vi "AutoDraw_Picture.vi"(7 "color(black)":u32(colorbox) caption="颜色（黑色）", 9 "Data Array for Picture":dbl[][](array[numeric]), 11 "Init Picture":picture) -> (2 "Anto Drawer":picture)   [LabVIEW 2014]
doc: "画平面图"
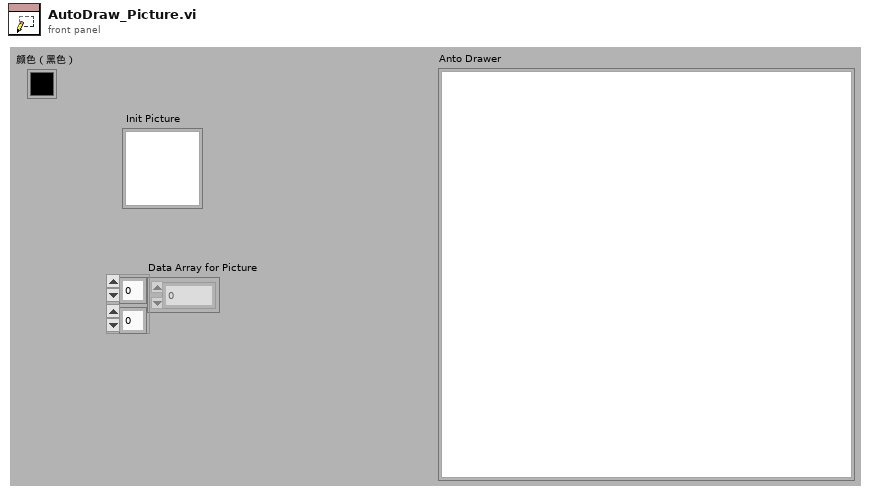
[diagram p1: front panel]
types:
  T1 = cluster{"Width":u16, "Style":enum32{"Solid", "Dash", "Dot", "DashDot", "DashDotDot"}}
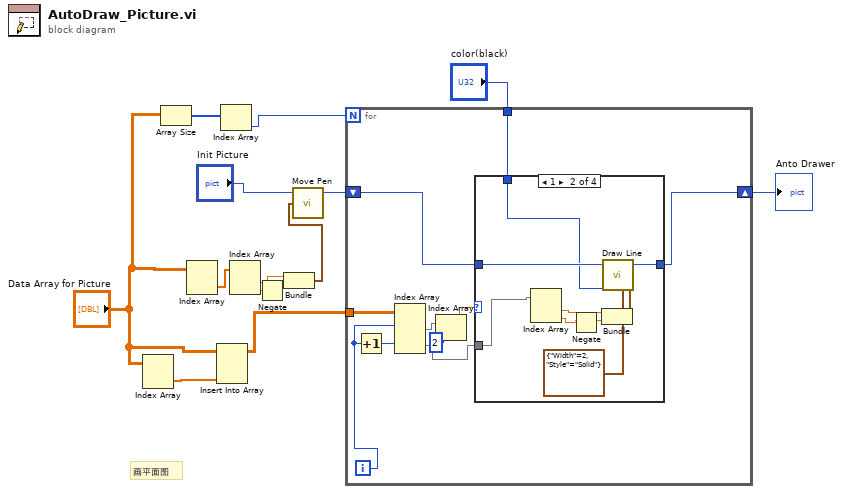
[diagram p0: block diagram]
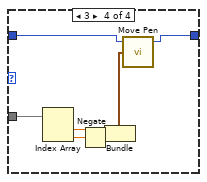
[diagram p4: hidden frame]
diagram:
  # "画平面图"
  n1 = Index Array(array="Data Array for Picture") -> (element=w7:dbl[])  [unwired: 2 in]
  n2 = Array Size(array="Data Array for Picture") -> (size(s)=w5:i32[])
  n3 = Index Array(array="Data Array for Picture") -> (element=w12:dbl[])  [unwired: 2 in]
  n4 = Insert Into Array(array="Data Array for Picture", new element=w7) -> (w6:dbl[][])  [unwired: 2 in]
  n5 = Index Array(array=w5) -> (element=w3:i32)  [unwired: 1 in]
  n6 = Index Array(array=w12) -> (element #1=w13:dbl, element #2=w14:dbl)  [unwired: 2 in]
  n7 = Negate(x=w14) -> (-x=w1:dbl)
  n8 = Bundle("x"=w13, w1) -> (w10:cluster{"x":dbl, dbl})  [unwired: 1 in]
  n9 = call <vilib>:"Move Pen.vi"("new position"=w10, "picture"="Init Picture") -> ("new picture"=w9:picture)  [unwired: 3 in]
  n10 = for {
    N: w3 -> [_]
    tunnel: w6 -> [w24]
    shift-right: [w16] -> w8
    shift-left: w9 -> [w20]
    tunnel: "color(black)" -> [w15]
    i -> [w18]
    n11 = Increment(x=w18) -> (x+1=w19:i32)
    n12 = Index Array(array=w24, index (row) #1=w18, index (row) #2=w19) -> (element #1=w21:dbl[], element #2=w17:dbl[])  [unwired: 2 in]
    n13 = Index Array(array=w21, index=2 ("索引")) -> (element=w22:dbl)
    n14 = case shown="1" w22 {
      tunnel: w20 -> [w25 w31 w35 w38]
      tunnel: [w25 w30 w35 w37] -> w16
      tunnel: w17 -> [_ w29 _ w40]
      tunnel: w15 -> [_ w27 _ _]
      frame 0, Default {
      }
      frame 1 {
        n15 = Index Array(array=w29) -> (element #1=w32:dbl, element #2=w33:dbl)  [unwired: 2 in]
        n16 = Negate(x=w33) -> (-x=w26:dbl)
        n17 = Bundle("x"=w32, w26) -> (w34:cluster{"x":dbl, dbl})  [unwired: 1 in]
        n18 = call <vilib>:"Draw Line.vi"("picture"=w31, "end point"=w34, "color(black)"=w27, "pen"=T1 {"Width"=2, "Style"=enum."Solid"}) -> ("new picture"=w30:picture)  [unwired: 5 in]
      }
      frame 2 {
      }
      frame 3 {
        n19 = Index Array(array=w40) -> (element #1=w41:dbl, element #2=w42:dbl)  [unwired: 2 in]
        n20 = Negate(x=w42) -> (-x=w36:dbl)
        n21 = Bundle("x"=w41, w36) -> (w39:cluster{"x":dbl, dbl})  [unwired: 1 in]
        n22 = call <vilib>:"Move Pen.vi"("new position"=w39, "picture"=w38) -> ("new picture"=w37:picture)  [unwired: 3 in]
      }
    }
  }
  "Anto Drawer" <- w8
